vi "CRYGet Max FSD In.vi"(6 "Signal Path":string[](array[string]), 8 "use ch name":bool, 9 "Wave in":T2[](array[typedef]) {"Y dB ref" format="%.1f"; "Y axis" items=["Log", "Lin"]; "Y data" items=["dB", "Lin"]; "X data" items=["dB", "Lin"]}, 10 "Max Level":dbl[](array[numeric]), 11 "Step No.":i32) -> (3 "Data Out":T1[](array[typedef]) {"Z data" items=["dB", "Lin"]; "X data" items=["dB", "Lin"]; "Y data" items=["dB", "Lin"]; "Z dB ref" format="%.1f"; "Z axis" items=["Log", "Lin"]; "X dB ref" format="%.1f"; "X axis" items=["Log", "Lin"]; "Y axis" items=["Log", "Lin"]; "Y dB ref" format="%.1f"; "Curve"."z" format="%.2f"; "Curve"."y" format="%.2f"; "Curve"."x" format="%.2f"})   [LabVIEW 2013]
uses:
  Typedef Control/CRYWaveform Cluster.ctl
  Typedef Control/CRYData Cluster.ctl
panel:
  in  "Acquisition Type":T3(ring)
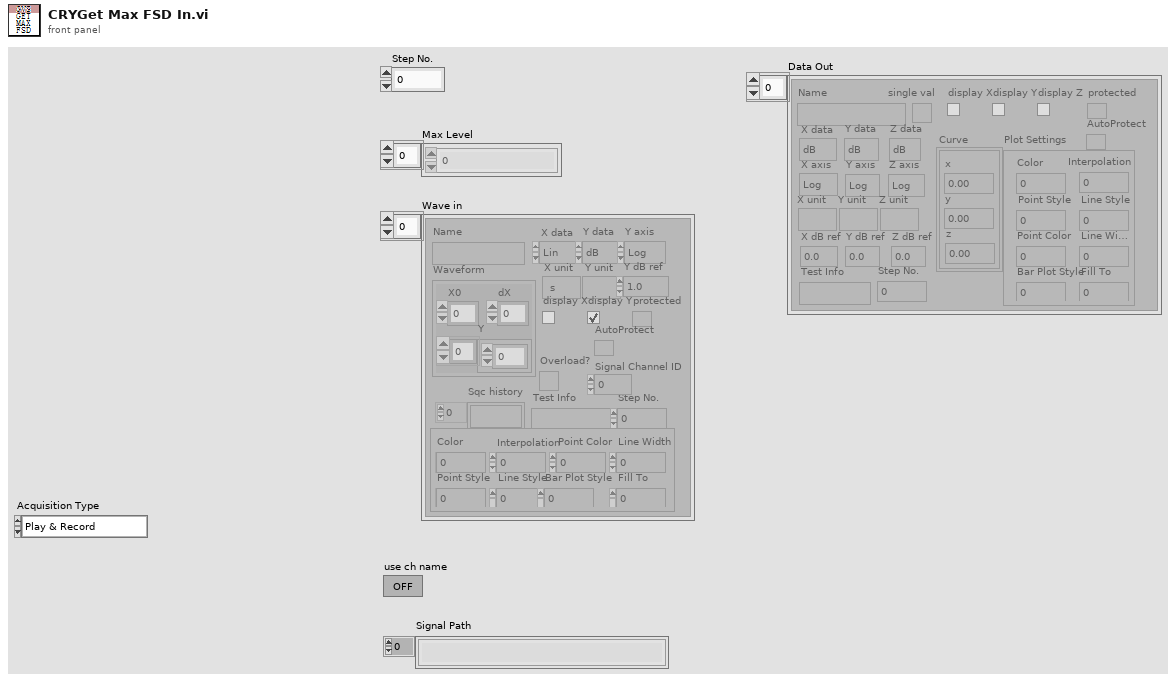
[diagram p1: front panel]
types:
  T1 = typedef "CRYData Cluster.ctl" = cluster{"Name":string, "Curve":cluster{"x":dbl, "y":dbl, "z":dbl}[], "X data":u16, "Y data":u16, "Z data":u16, "X axis":u16, "Y axis":u16, "Z axis":u16, "X unit":string, "Y unit":string, "Z unit":string, "X dB ref":dbl, "Y dB ref":dbl, "Z dB ref":dbl, "single val":bool, "protected":bool, "display X":bool, "display Y":bool, "display Z":bool, "Test Info":string, "Step No.":i32, "Plot Settings":cluster{"Color":u32, "Interpolation":u8, "Point Style":u8, "Line Style":u8, "Point Color":u32, "Line Width":u8, "Bar Plot Style":u8, "Fill To":i16}, "AutoProtect":bool}
  T2 = typedef "CRYWaveform Cluster.ctl" = cluster{"Waveform":cluster{"X0":dbl, "dX":dbl, "Y":sgl[]}, "X data":u16, "Y data":u16, "Y axis":u16, "X unit":string, "Y unit":string, "Y dB ref":dbl, "display Y":bool, "display X":bool, "Overload?":bool, "Test Info":string, "Step No.":i32, "Name":string, "protected":bool, "Sqc history":string[], "Signal Channel ID":i32, "Plot Settings":cluster{"Color":u32, "Interpolation":u8, "Point Style":u8, "Line Style":u8, "Point Color":u32, "Line Width":u8, "Bar Plot Style":u8, "Fill To":i16}, "AutoProtect":bool}
  T3 = enum16{"Play & Record", "Record", "Sine Generator", "Voltmeter", "Oscilloscope", "Spectrum Analyzer", "RTA", "Generator & Voltmeter", "Generator & Oscilloscope", "Generator & Spectrum", "Generator & RTA", "Read From DC Connect"}
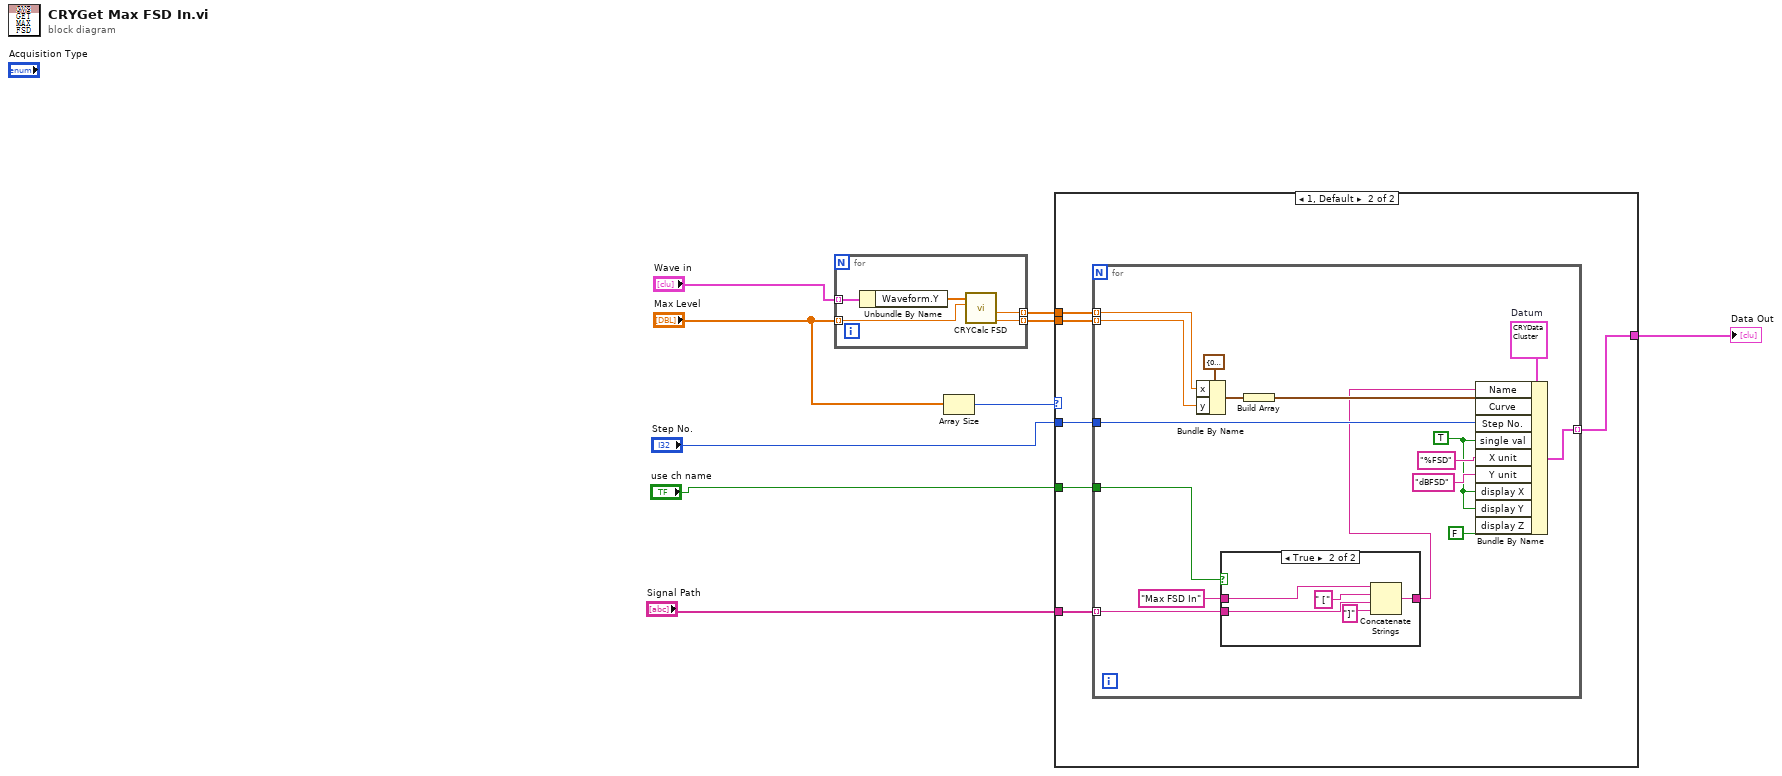
[diagram p0: block diagram]
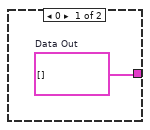
[diagram p2: hidden frame]
diagram:
  n1 = for {
    tunnel: "Wave in" -> [w14] mode=indexing
    tunnel: [w12] -> w8 mode=indexing
    tunnel: [w11] -> w7 mode=indexing
    tunnel: "Max Level" -> [w10] mode=indexing
    n2 = Unbundle By Name(w14) -> ("Waveform.Y"=w13:sgl[])
    n3 = call "CRYCalc FSD.vi"("Max Level"=w10, "X"=w13) -> ("dBFSD(RMS)"=w11:dbl, "%FSD(RMS)"=w12:dbl)  [unwired: 6 in, 2 out]
  }
  n4 = Array Size(array="Max Level") -> (size(s)=w9:i32)
  n5 = case shown="1, Default" w9 {
    tunnel: "Step No." -> [_ w21]
    tunnel: w8 -> [_ w20]
    tunnel: w7 -> [_ w19]
    tunnel: [w15 w18] -> w6
    tunnel: "use ch name" -> [_ w17]
    tunnel: "Signal Path" -> [_ w16]
    frame 0 {
      w15 = T1[] []  # Data Out
    }
    frame 1, Default {
      n6 = for {
        tunnel: w21 -> [w31]
        tunnel: w20 -> [w30] mode=indexing
        tunnel: w19 -> [w29] mode=indexing
        tunnel: [w28] -> w18 mode=indexing
        tunnel: w17 -> [w27]
        tunnel: w16 -> [w25] mode=indexing
        w37 = T1 {"Name"="", "Curve"=[], "X data"=1, "Y data"=1, "Z data"=1, "X axis"=0, "Y axis"=1, "Z axis"=1, "X unit"="Hz", "Y unit"="", "Z unit"="deg.", "X dB ref"=1.0, "Y dB ref"=1.0, "Z dB ref"=1.0, "single val"=FALSE, "protected"=FALSE, "display X"=TRUE, "display Y"=TRUE, "display Z"=FALSE, "Test Info"="", "Step No."=0, "Plot Settings"={"Color"=0, "Interpolation"=0, "Point Style"=0, "Line Style"=0, "Point Color"=0, "Line Width"=0, "Bar Plot Style"=0, "Fill To"=0}, "AutoProtect"=FALSE}  # Datum
        w23 = TRUE ("single val")
        n7 = Bundle By Name(cluster=cluster{"x":dbl, "y":dbl, "z":dbl} {"x"=0.0, "y"=0.0, "z"=0.0}, "x"=w30, "y"=w29) -> (w35:cluster{"x":dbl, "y":dbl, "z":dbl})
        n8 = case shown="True" w27 {
          tunnel: "Max FSD In" ("Name") -> [w38 w41]
          tunnel: [w38 w40] -> w24
          tunnel: w25 -> [_ w39]
          frame False {
          }
          frame True {
            n9 = Concatenate Strings(w41, " [" ("string"), w39, "]" ("string")) -> (w40:string)
          }
        }
        n10 = Build Array(w35) -> (w34:cluster{"x":dbl, "y":dbl, "z":dbl}[])
        n11 = Bundle By Name(cluster=w37, "Name"=w24, "Curve"=w34, "Step No."=w31, "single val"=w23, "X unit"="%FSD", "Y unit"="dBFSD", "display X"=w23, "display Y"=w23, "display Z"=FALSE ("single val")) -> (w28:T1)
      }
    }
  }
  "Data Out" <- w6
